vi "DCV_CheckStart.vi"(6 "LowLimit":dbl, 7 "HiLimit":dbl, 8 "Error In":errorcluster, 10 "channel":string="116", 11 "VISA resource name":refnum<visa-resource-name>="COM5") -> (0 "Error Out":errorcluster, 2 "value":dbl, 3 "VISA resource name out":refnum<visa-resource-name>="COM5")   [LabVIEW 2013]
uses:
  <vilib>/Utility/error.llb/whitespace.ctl
panel:
  out "testlist":dbl[](array[numeric])=[1.33831, 1.33831, 1.33831, 1.33831, 1.3383, 1.3383, 1.3383, 1.3383, 1.33829, 1.33829, 1.33829, 1.33829, 1.33828, 1.33828, 1.33828, 1.33828]
  out "read buffer 2":string="SCAN OK\n"
  out "Value":string
  out "Array":dbl[](array[numeric])
  out "read buffer":string="SCAN OK\n"
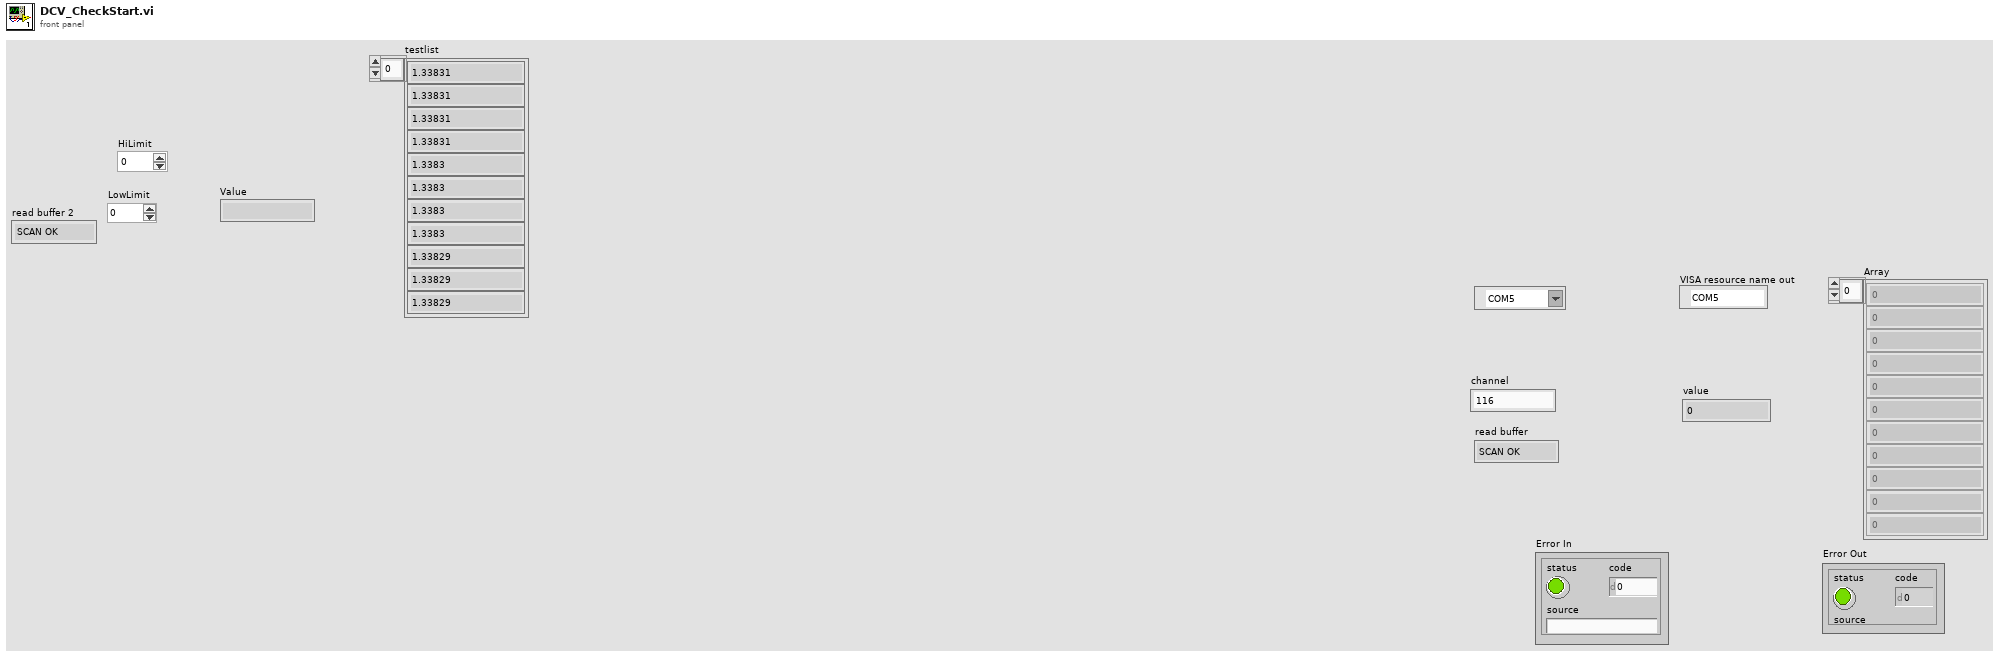
[diagram p1: front panel]
types:
  T1 = typedef "whitespace.ctl" = u16
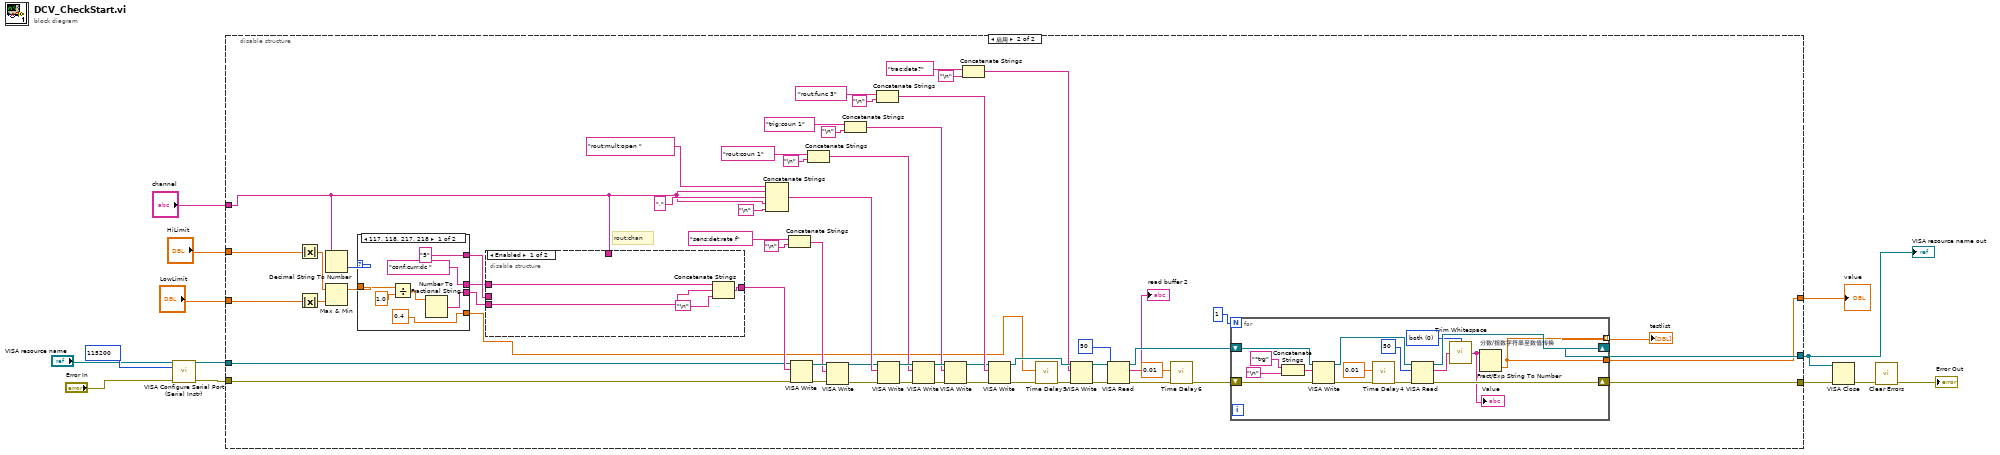
[diagram p0: block diagram]
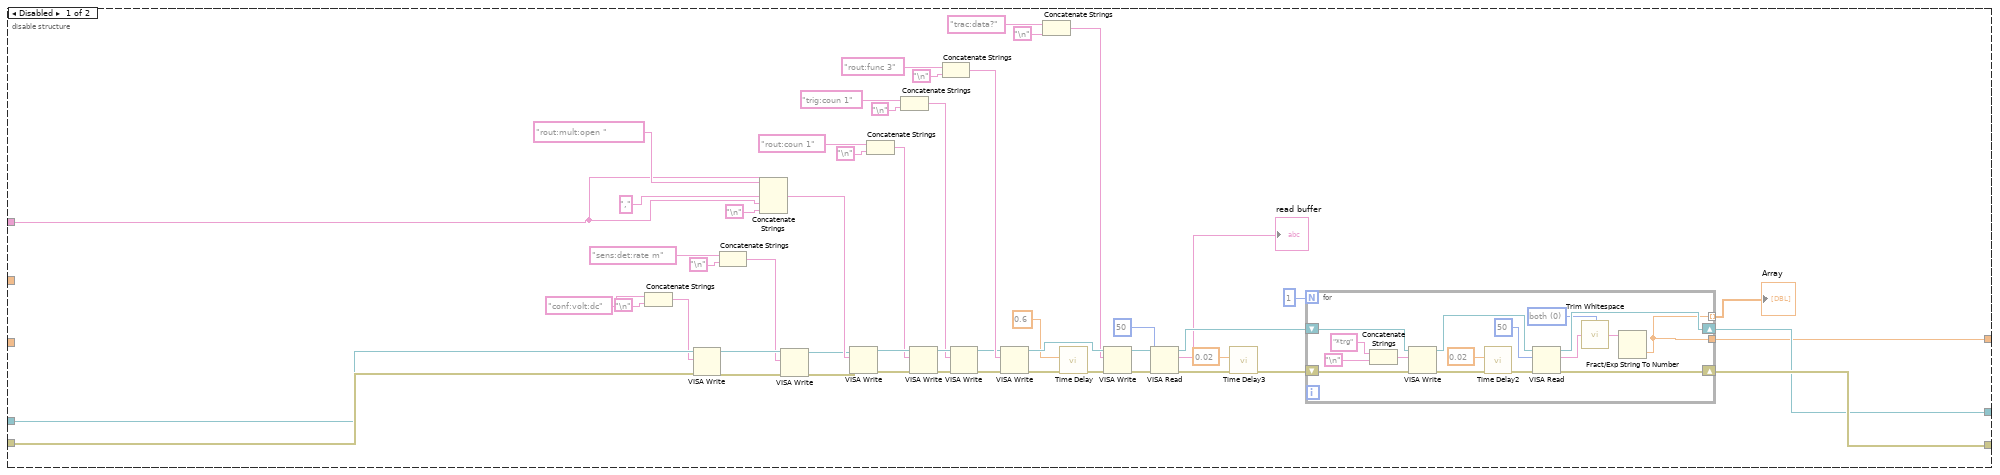
[diagram p2: hidden frame]
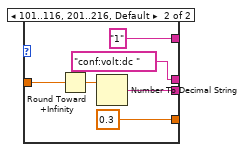
[diagram p3: hidden frame]
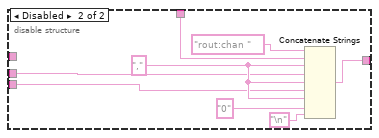
[diagram p4: hidden frame]
diagram:
  n1 = call <vilib>:"VISA Configure Serial Port (Serial Instr).vi"("VISA resource name"="VISA resource name", "baud rate (9600)"=u32 115200, "error in (no error)"="Error In") -> ("VISA resource name out"=w4:refnum<visa-resource-name>, "error out"=w13:errorcluster)  [unwired: 11 in]
  n2 = disable-structure shown="启用" {
    disable-tunnel: w13 -> [w65 w88]
    disable-tunnel: w4 -> [w64 w87]
    disable-tunnel: [w63 w86] -> w12
    disable-tunnel: [w62 w85] -> w3
    disable-tunnel: "channel" -> [w23 w89]
    disable-tunnel: "LowLimit" -> [_ w84]
    disable-tunnel: "HiLimit" -> [_ w83]
    disable-tunnel: [w14 w82] -> w8
    frame Disabled {
      n3 = Concatenate Strings("conf:volt:dc" ("write buffer"), "\n") -> (w59:string)
      n4 = VISA Write(VISA resource name=w64, write buffer=w59, error in (no error)=w65) -> (VISA resource name out=w17:refnum<visa-resource-name>, error out=w18:errorcluster)  [unwired: 1 out]
      n5 = Concatenate Strings("sens:det:rate m" ("write buffer"), "\n") -> (w15:string)
      n6 = Concatenate Strings("rout:mult:open ", w23, ",", w23, "\n") -> (w58:string)
      n7 = VISA Write(VISA resource name=w17, write buffer=w15, error in (no error)=w18) -> (VISA resource name out=w16:refnum<visa-resource-name>, error out=w19:errorcluster)  [unwired: 1 out]
      n8 = VISA Write(VISA resource name=w16, write buffer=w58, error in (no error)=w19) -> (VISA resource name out=w56:refnum<visa-resource-name>, error out=w57:errorcluster)  [unwired: 1 out]
      n9 = Concatenate Strings("rout:coun 1" ("write buffer"), "\n") -> (w53:string)
      n10 = Concatenate Strings("trig:coun 1" ("write buffer"), "\n") -> (w48:string)
      n11 = VISA Write(VISA resource name=w56, write buffer=w53, error in (no error)=w57) -> (VISA resource name out=w51:refnum<visa-resource-name>, error out=w52:errorcluster)  [unwired: 1 out]
      n12 = Concatenate Strings("rout:func 3" ("write buffer"), "\n") -> (w45:string)
      n13 = VISA Write(VISA resource name=w51, write buffer=w48, error in (no error)=w52) -> (VISA resource name out=w24:refnum<visa-resource-name>, error out=w25:errorcluster)  [unwired: 1 out]
      n14 = VISA Write(VISA resource name=w24, write buffer=w45, error in (no error)=w25) -> (VISA resource name out=w43:refnum<visa-resource-name>, error out=w44:errorcluster)  [unwired: 1 out]
      n15 = Concatenate Strings("trac:data?" ("write buffer"), "\n") -> (w34:string)
      n16 = call "Time Delay"("error in (no error)"=w44, "Delay Time (s)"=0.6 ("wait scan")) -> ("error out"=w33:errorcluster)  [unwired: 9 in]
      n17 = VISA Write(VISA resource name=w43, write buffer=w34, error in (no error)=w33) -> (VISA resource name out=w31:refnum<visa-resource-name>, error out=w32:errorcluster)  [unwired: 1 out]
      n18 = VISA Read(VISA resource name=w31, byte count=u32 50, error in (no error)=w32) -> (VISA resource name out=w41:refnum<visa-resource-name>, read buffer=→"read buffer":string, error out=w27:errorcluster)  [unwired: 1 out]
      n19 = call "Time Delay3"("error in (no error)"=w27, "Delay Time (s)"=0.02) -> ("error out"=w42:errorcluster)  [unwired: 9 in]
      n20 = for {
        N: 1 -> [_]
        shift-right: [w81] -> w63
        shift-left: w42 -> [w71]
        shift-right: [w80] -> w62
        shift-left: w41 -> [w70]
        tunnel: [w66] -> w22 mode=indexing
        tunnel: [w66] -> w14
        w68 = T1 0 items=["both", "start of string", "end of string"] ("location (both)")
        n21 = Concatenate Strings("*trg" ("write buffer"), "\n") -> (w76:string)
        n22 = VISA Write(VISA resource name=w70, write buffer=w76, error in (no error)=w71) -> (VISA resource name out=w73:refnum<visa-resource-name>, error out=w75:errorcluster)  [unwired: 1 out]
        n23 = call "Time Delay2"("error in (no error)"=w75, "Delay Time (s)"=0.02) -> ("error out"=w74:errorcluster)  [unwired: 9 in]
        n24 = VISA Read(VISA resource name=w73, byte count=u32 50, error in (no error)=w74) -> (VISA resource name out=w80:refnum<visa-resource-name>, read buffer=w69:string, error out=w81:errorcluster)  [unwired: 1 out]
        n25 = call <vilib>:"Trim Whitespace.vi"("string"=w69, "location (both)"=w68) -> ("trimmed string"=w67:string)
        n26 = Fract/Exp String To Number(string=w67) -> (number=w66:dbl)  [unwired: 3 in, 1 out]
      }
      "Array" <- w22
    }
    frame Enabled {
      # "rout:chan"
      n27 = Absolute Value(x=w83) -> (abs(x)=w101:dbl)
      n28 = Absolute Value(x=w84) -> (abs(x)=w102:dbl)
      n29 = Decimal String To Number(string=w89) -> (number=w103:i32)  [unwired: 2 in, 1 out]
      n30 = Max & Min(x=w101, y=w102) -> (max(x,y)=w100:dbl)  [unwired: 1 out]
      n31 = case shown="117, 118, 217, 218" w103 {
        tunnel: ["5" "1"] -> w104
        tunnel: w100 -> [w145 w151]
        tunnel: [w142 w150] -> w99
        tunnel: ["conf:curr:dc " ("write buffer") "conf:volt:dc " ("write buffer")] -> w98
        tunnel: [0.4 ("wait scan") 0.3 ("wait scan")] -> w90
        frame 117, 118, 217, 218 {
          n32 = Divide(x=w145, y=1.0) -> (x/y=w143:dbl)
          n33 = Number To Fractional String(number=w143) -> (F-format string=w142:string)  [unwired: 3 in]
        }
        frame 101..116, 201..216, Default {
          n34 = Round Toward +Infinity(x=w151) -> (ceil(x): smallest int >= x=w152:dbl)
          n35 = Number To Decimal String(number=w152) -> (decimal integer string=w150:string)  [unwired: 1 in]
        }
      }
      n36 = disable-structure shown="Enabled" {
        disable-tunnel: [w157 w163] -> w140
        disable-tunnel: w89 -> [_ w164]
        disable-tunnel: w104 -> [_ w159]
        disable-tunnel: w99 -> [w156 w158]
        disable-tunnel: w98 -> [w154 _]
        frame Enabled {
          n37 = Concatenate Strings(w154, w156, "\n") -> (w157:string)
        }
        frame Disabled {
          w162 = ","
          n38 = Concatenate Strings("rout:chan " ("write buffer"), w164, w162, w159, w162, w158, w162, "0" ("string"), "\n") -> (w163:string)
        }
      }
      n39 = Concatenate Strings("rout:mult:open ", w89, ",", w89, "\n") -> (w139:string)
      n40 = Concatenate Strings("sens:det:rate f" ("write buffer"), "\n") -> (w91:string)
      n41 = VISA Write(VISA resource name=w87, write buffer=w140, error in (no error)=w88) -> (VISA resource name out=w96:refnum<visa-resource-name>, error out=w97:errorcluster)  [unwired: 1 out]
      n42 = Concatenate Strings("rout:coun 1" ("write buffer"), "\n") -> (w134:string)
      n43 = VISA Write(VISA resource name=w96, write buffer=w91, error in (no error)=w97) -> (VISA resource name out=w94:refnum<visa-resource-name>, error out=w95:errorcluster)  [unwired: 1 out]
      n44 = Concatenate Strings("trig:coun 1" ("write buffer"), "\n") -> (w129:string)
      n45 = Concatenate Strings("rout:func 3" ("write buffer"), "\n") -> (w126:string)
      n46 = VISA Write(VISA resource name=w94, write buffer=w139, error in (no error)=w95) -> (VISA resource name out=w137:refnum<visa-resource-name>, error out=w138:errorcluster)  [unwired: 1 out]
      n47 = VISA Write(VISA resource name=w137, write buffer=w134, error in (no error)=w138) -> (VISA resource name out=w132:refnum<visa-resource-name>, error out=w133:errorcluster)  [unwired: 1 out]
      n48 = VISA Write(VISA resource name=w132, write buffer=w129, error in (no error)=w133) -> (VISA resource name out=w106:refnum<visa-resource-name>, error out=w107:errorcluster)  [unwired: 1 out]
      n49 = Concatenate Strings("trac:data?" ("write buffer"), "\n") -> (w115:string)
      n50 = VISA Write(VISA resource name=w106, write buffer=w126, error in (no error)=w107) -> (VISA resource name out=w124:refnum<visa-resource-name>, error out=w125:errorcluster)  [unwired: 1 out]
      n51 = call "Time Delay5"("error in (no error)"=w125, "Delay Time (s)"=w90) -> ("error out"=w114:errorcluster)  [unwired: 9 in]
      n52 = VISA Write(VISA resource name=w124, write buffer=w115, error in (no error)=w114) -> (VISA resource name out=w112:refnum<visa-resource-name>, error out=w113:errorcluster)  [unwired: 1 out]
      n53 = VISA Read(VISA resource name=w112, byte count=u32 50, error in (no error)=w113) -> (VISA resource name out=w122:refnum<visa-resource-name>, read buffer=→"read buffer 2":string, error out=w109:errorcluster)  [unwired: 1 out]
      n54 = call "Time Delay6"("error in (no error)"=w109, "Delay Time (s)"=0.01) -> ("error out"=w123:errorcluster)  [unwired: 9 in]
      n55 = for {
        N: 1 -> [_]
        shift-right: [w181] -> w86
        shift-left: w123 -> [w171]
        shift-right: [w180] -> w85
        shift-left: w122 -> [w170]
        tunnel: [w166] -> w105 mode=indexing
        tunnel: [w166] -> w82
        w168 = T1 0 items=["both", "start of string", "end of string"] ("location (both)")
        n56 = Concatenate Strings("*trg" ("write buffer"), "\n") -> (w176:string)
        n57 = VISA Write(VISA resource name=w170, write buffer=w176, error in (no error)=w171) -> (VISA resource name out=w173:refnum<visa-resource-name>, error out=w175:errorcluster)  [unwired: 1 out]
        n58 = call "Time Delay4"("error in (no error)"=w175, "Delay Time (s)"=0.01) -> ("error out"=w174:errorcluster)  [unwired: 9 in]
        n59 = VISA Read(VISA resource name=w173, byte count=u32 50, error in (no error)=w174) -> (VISA resource name out=w180:refnum<visa-resource-name>, read buffer=w169:string, error out=w181:errorcluster)  [unwired: 1 out]
        n60 = call <vilib>:"Trim Whitespace.vi"("string"=w169, "location (both)"=w168) -> ("trimmed string"=w167:string)
        "Value" <- w167
        n61 = Fract/Exp String To Number "分数/指数字符串至数值转换"(string=w167) -> (number=w166:dbl)  [unwired: 3 in, 1 out]
      }
      "testlist" <- w105
    }
  }
  "VISA resource name out" <- w3
  "value" <- w8
  n62 = VISA Close(VISA resource name=w3, error in (no error)=w12) -> (error out=w2:errorcluster)
  n63 = call <vilib>:"Clear Errors.vi"("error in (no error)"=w2) -> ("error out"=→"Error Out":errorcluster)  [unwired: 6 in]
